vi "Actor Core.vi"(8 "error in":errorcluster, 11 "LF2R IDE in":refnum<class "Main Panel.lvclass">) -> (0 "error out":errorcluster, 3 "Actor out":refnum<class "Actor.lvclass">)   [LabVIEW 2018, in "Main Panel.lvlib" / "Main Panel.lvclass"]
doc: "The user interface for this panel.\n\n----\nPlease see the following web address for additional documentation and tutorial information:\nhttp://www.mooregoodideas.com/mgi-panel-manager/\n\nAuthor: Derek Trepanier\n\nCopyright (c) 2018, Moore Good Ideas, Inc.\n\nAll rights reserved.\n\nRedistribution and use in source and binary forms, with or without modification, are permitted provided that the following conditions are met:\n\n * Redistributions of source code must retain the above copyright notice, this list of conditions and the following disclaimer.\n * Redistributions in binary form must reproduce the above copyright notice, this list of conditions and the following disclaimer in the documentation and/or other materials provided with the distribution.\n * Neither the name of Moore Good Ideas, Inc. nor the names of its contributors may be used to endorse or promote products derived from this software without specific prior written permission.\n\nTHIS SOFTWARE IS PROVIDED BY THE COPYRIGHT HOLDERS AND CONTRIBUTORS \"AS IS\" AND ANY EXPRESS OR IMPLIED WARRANTIES, INCLUDING, BUT NOT LIMITED TO, THE IMPLIED WARRANTIES OF MERCHANTABILITY AND FITNESS FOR A PARTICULAR PURPOSE ARE DISCLAIMED. IN NO EVENT SHALL THE COPYRIGHT OWNER OR CONTRIBUTORS BE LIABLE FOR ANY DIRECT, INDIRECT, INCIDENTAL, SPECIAL, EXEMPLARY, OR CONSEQUENTIAL DAMAGES (INCLUDING, BUT NOT LIMITED TO, PROCUREMENT OF SUBSTITUTE GOODS OR SERVICES; LOSS OF USE, DATA, OR PROFITS; OR BUSINESS INTERRUPTION) HOWEVER CAUSED AND ON ANY THEORY OF LIABILITY, WHETHER IN CONTRACT, STRICT LIABILITY, OR TORT (INCLUDING NEGLIGENCE OR OTHERWISE) ARISING IN ANY WAY OUT OF THE USE OF THIS SOFTWARE, EVEN IF ADVISED OF THE POSSIBILITY OF SUCH DAMAGE."
uses:
  Main Panel.lvclass
  C:/Program Files (x86)/National Instruments/LabVIEW 2018/vi.lib/MGI/Panel Manager/Panel Actor/Panel Actor/Panel Actor.lvclass
  <vilib>/ActorFramework/Actor/Actor.lvclass
  Main Panel.lvclass/Main Panel.ctl
  Const Configuration.ctl
  Const Path Setting.ctl
  Const Image Viewer Setting.ctl
  Framework/Framework/Framework.lvclass
  <vilib>/MGI/Panel Manager/Panel Actor/Panel Actor/Panel Actor.lvclass
  D:/project/hobby/LabVIEW/LF2R/LabVIEW/Source/ScintillaNET/dll/ScintillaNET.dll
  ScintillaNET/dll/ScintillaNET.dll
panel:
  in  "File Path":path
  in  "Script":refnum<k24>(container)
  in  "To Next Frame":bool
  in  "Go to Frame":u16(ring)
  in  "Tab Control":T1(tab)
  in  "WindowsMediaPlayer":refnum<k7>(container)
  in  "basic_state":u16(ring) caption="state" items=["Stand"=0, "Walk"=1, "Run"=2, "Attacking"=3, "Jumping"=4, "Dashing"=5, "Rowing"=6, "Defending"=7, "Defend Broken"=8, "Catching"=9, "Caught"=10, "Injured"=11, "Falling"=12, "Ice"=13, "Lying"=14, "Normal"=15, "Faint"=16, "Drinking"=17, "Burning (Can Attack Teammate)"=18, "Burning Run"=19, "Louis's Special Landing (to frame 94)"=100, "Deep's Special Move (Can Control Up and Down)"=301, "Teleport to the Nearest Teammate"=400, "Teleport to the Nearest Enemy"=401, "Rudolf's Transform"=500, "Rudolf's Transform Back"=501, "Healing"=1700, "Transform to ID (80XX, ID: XX)"=8000, "Transform to LouisEx"=9995, "Message"=9997, "Message Delete"=9998, "Broken Weapon"=9999]
  in  "sound":string
  in  "basic_dvz":i32 caption="dvz"
  in  "basic_dvy":i32 caption="dvy"
  in  "basic_dvx":i32 caption="dvx"
  in  "basic_centery":i32 caption="centery"
  in  "basic_centerx":i32 caption="centerx"
  in  "basic_next":u32 caption="next"
  in  "basic_wait":u32 caption="wait"
  in  "basic_pic":u32 caption="pic"
  in  "basic_mp":i32 caption="mp"
  in  "basic_hit_j":u32 caption="hit_j"
  in  "basic_hit_a":u32 caption="hit_a"
  in  "basic_hit_d":u32 caption="hit_d"
  in  "basic_hit_ja":u32 caption="hit_ja"
  in  "basic_hit_Ua":u32 caption="hit_Ua"
  in  "basic_hit_Fa":u32 caption="hit_Fa"
  in  "basic_hit_Da":u32 caption="hit_Da"
  in  "basic_hit_Dj":u32 caption="hit_Dj"
  in  "basic_hit_Uj":u32 caption="hit_Uj"
  in  "basic_hit_Fj":u32 caption="hit_Fj"
  in  "Sound Play":bool caption="Play"
  in  "bp_y":dbl caption="y"
  in  "bp_x":dbl caption="x"
  in  "w_attacking":u32 caption="attacking"
  in  "w_dvz":i32 caption="dvz"
  in  "w_dvy":i32 caption="dvy"
  in  "w_dvx":i32 caption="dvx"
  in  "w_cover":u32 caption="cover"
  in  "w_weaponact":u32 caption="weaponact"
  in  "w_y":dbl caption="y"
  in  "w_x":dbl caption="x"
  in  "w_kind":u32 caption="kind"
  in  "b_h":u32 caption="h"
  in  "b_w":u32 caption="w"
  in  "b_y":i32 caption="y"
  in  "b_x":i32 caption="x"
  in  "b_kind":u32 caption="kind"
  in  "<b> index":u32(slide) scale=0.0..10.0
  in  "i_zwidth":u32 caption="zwidth"
  in  "i_caughtact 2":u32 caption="caughtact 2"
  in  "i_catchingact 2":u32 caption="catchingact 2"
  in  "i_caughtact 1":u32 caption="caughtact 1"
  in  "i_catchingact 1":u32 caption="catchingact 1"
  in  "i_effect":u32 caption="effect"
  in  "i_injury":i32 caption="injury"
  in  "i_bdefend":i32 caption="bdefend"
  in  "i_vrest":u32 caption="vrest"
  in  "i_arest":u32 caption="arest"
  in  "i_fall":u32 caption="fall"
  in  "i_dvz":i32 caption="dvz"
  in  "i_dvy":i32 caption="dvy"
  in  "i_dvx":i32 caption="dvx"
  in  "i_h":u32 caption="h"
  in  "i_w":u32 caption="w"
  in  "i_y":i32 caption="y"
  in  "i_x":i32 caption="x"
  in  "i_kind":u32 caption="kind"
  in  "<i> index":u32(slide) scale=0.0..10.0
  in  "o_facing":i32 caption="facing"
  in  "o_oid":u32 caption="oid"
  in  "o_action":u32 caption="action"
  in  "o_kind":u32 caption="kind"
  in  "o_x":i32 caption="x"
  in  "o_y":i32 caption="y"
  in  "o_dvx":i32 caption="dvx"
  in  "o_dvy":i32 caption="dvy"
  in  "o_dvz":i32 caption="dvz"
  in  "c_cover":i32 caption="cover"
  in  "c_injury":i32 caption="injury"
  in  "c_dircontrol":i32 caption="dircontrol"
  in  "c_backhurtact":i32 caption="backhurtact"
  in  "c_fronthurtact":i32 caption="fronthurtact"
  in  "c_decrease":i32 caption="decrease"
  in  "c_hurtable":i32 caption="hurtable"
  in  "c_taction":i32 caption="taction"
  in  "c_aaction":i32 caption="aaction"
  in  "c_vaction":i32 caption="vaction"
  in  "c_y":i32 caption="y"
  in  "c_x":i32 caption="x"
  in  "c_kind":u32 caption="kind"
  in  "c_throwvx":i32 caption="throwvx"
  in  "c_throwvy":i32 caption="throwvy"
  in  "c_throwvz":i32 caption="throwvz"
  in  "c_throwinjury":i32 caption="throwinjury"
  in  "title_name":string caption="Name"
  in  "Apply Change":bool
  in  "title_num":u32 caption="Frame Num" format="%03d"
  out "Picture":picture
  out "String":string
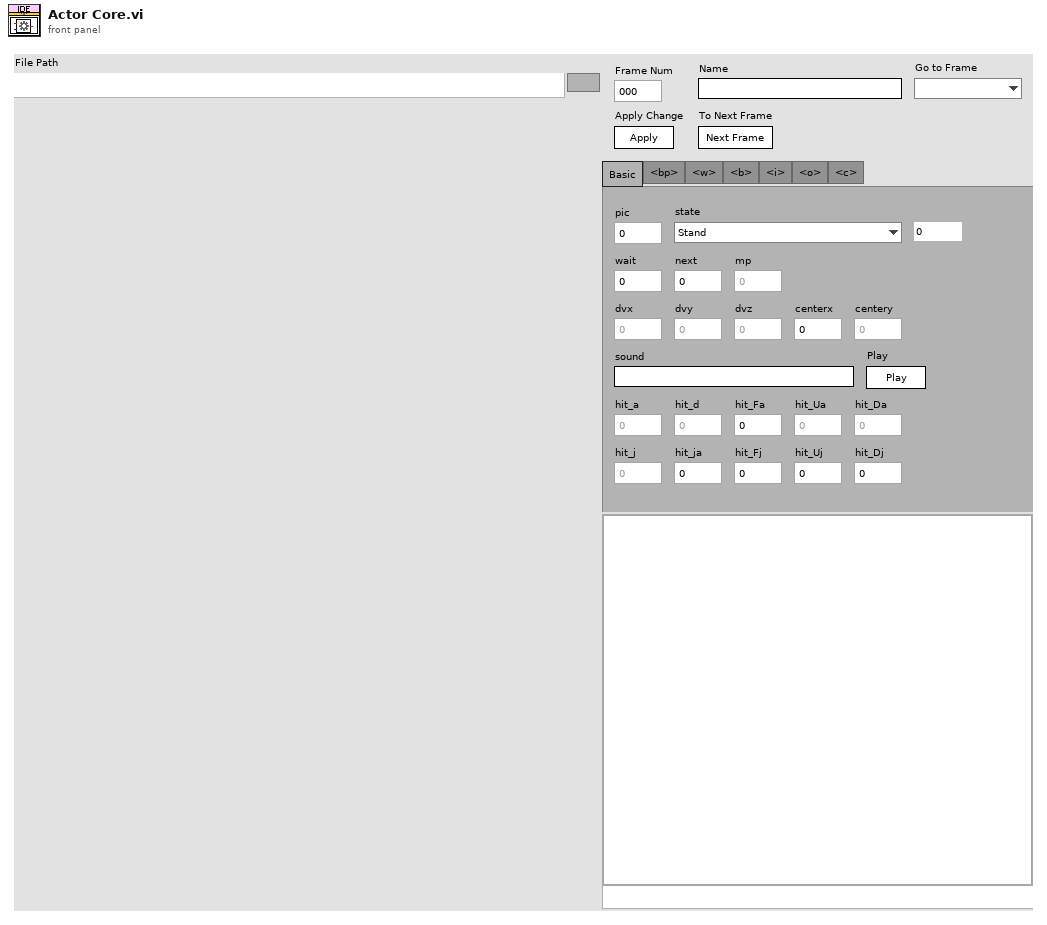
[diagram p1: front panel]
types:
  T1 = enum32{"Basic", "<bp>", "<w>", "<b>", "<i>", "<o>", "<c>"}
  T2 = cluster{"title_num":refnum<vi>, "title_name":refnum<vi>}
  T3 = cluster{"basic_pic":refnum<vi>, "basic_state":refnum<vi>, "basic_wait":refnum<vi>, "basic_next":refnum<vi>}
  T4 = cluster{"basic_centerx":refnum<vi>, "basic_centery":refnum<vi>}
  T5 = cluster{"basic_dvx":refnum<vi>, "basic_dvy":refnum<vi>, "basic_dvz":refnum<vi>}
  T6 = cluster{"b_kind":refnum<vi>, "b_x":refnum<vi>, "b_y":refnum<vi>, "b_w":refnum<vi>, "b_h":refnum<vi>, "<b> index":refnum<vi>}
  T7 = cluster{"w_kind":refnum<vi>, "w_x":refnum<vi>, "w_y":refnum<vi>, "w_weaponact":refnum<vi>, "w_dvx":refnum<vi>, "w_dvy":refnum<vi>, "w_dvz":refnum<vi>, "w_attacking":refnum<vi>, "w_cover":refnum<vi>}
  T8 = cluster{"basic_hit_a":refnum<vi>, "basic_hit_d":refnum<vi>, "basic_hit_j":refnum<vi>, "basic_hit_Fa":refnum<vi>, "basic_hit_Ua":refnum<vi>, "basic_hit_Da":refnum<vi>, "basic_hit_Fj":refnum<vi>, "basic_hit_Uj":refnum<vi>, "basic_hit_Dj":refnum<vi>, "basic_hit_ja":refnum<vi>}
  T9 = cluster{"o_kind":refnum<vi>, "o_x":refnum<vi>, "o_y":refnum<vi>, "o_action":refnum<vi>, "o_dvx":refnum<vi>, "o_dvy":refnum<vi>, "o_dvz":refnum<vi>, "o_oid":refnum<vi>, "o_facing":refnum<vi>}
  T10 = cluster{"i_kind":refnum<vi>, "i_x":refnum<vi>, "i_y":refnum<vi>, "i_w":refnum<vi>, "i_h":refnum<vi>, "i_dvx":refnum<vi>, "i_dvy":refnum<vi>, "i_dvz":refnum<vi>, "i_fall":refnum<vi>, "i_arest":refnum<vi>, "i_vrest":refnum<vi>, "i_bdefend":refnum<vi>, "i_injury":refnum<vi>, "i_zwidth":refnum<vi>, "i_effect":refnum<vi>, "i_catchingact 1":refnum<vi>, "i_catchingact 2":refnum<vi>, "i_caughtact 1":refnum<vi>, "i_caughtact 2":refnum<vi>, "<i> index":refnum<vi>}
  T11 = cluster{"c_kind":refnum<vi>, "c_x":refnum<vi>, "c_y":refnum<vi>, "c_injury":refnum<vi>, "c_cover":refnum<vi>, "c_vaction":refnum<vi>, "c_aaction":refnum<vi>, "c_taction":refnum<vi>, "c_hurtable":refnum<vi>, "c_decrease":refnum<vi>, "c_fronthurtact":refnum<vi>, "c_backhurtact":refnum<vi>, "c_dircontrol":refnum<vi>, "c_throwvx":refnum<vi>, "c_throwvy":refnum<vi>, "c_throwvz":refnum<vi>, "c_throwinjury":refnum<vi>}
  T12 = cluster{"Event Registration Refnum":refnum<event-registration>, "Pnl Actor":refnum<event-registration>}
  T13 = typedef "Main Panel.lvlib/Main Panel.lvclass/Const Configuration.ctl" = cluster{"Language":cluster{"Name":string}, "Path Config":T14, "Image Viewer Config":T15}
  T14 = typedef "Main Panel.lvlib/Main Panel.lvclass/Const Path Setting.ctl" = cluster{"Data Folder Path":path, "PNG Folder Path":path, "mp3 Folder Path":path}
  T15 = typedef "Main Panel.lvlib/Main Panel.lvclass/Const Image Viewer Setting.ctl" = cluster{"Center Point":cluster{"Size":i32, "Color":u32, "Show?":bool}, "bp Point":cluster{"Size":i32, "Color":u32, "Show?":bool}, "w Point":cluster{"Size":i32, "Color":u32, "Show?":bool}, "b Box":cluster{"Fill Color":u32, "Border Color":u32, "Show?":bool}, "i Box":cluster{"Fill Color":u32, "Border Color":u32, "Show?":bool}, "o Point":cluster{"Size":i32, "Color":u32, "Show?":bool}, "c Point":cluster{"Size":i32, "Color":u32, "Show?":bool}}
  T16 = typedef "LF2R IDE.lvlib/LF2R IDE.lvclass/LF2R IDE Cmd.ctl" = enum16{"Save Data File", "Write Configuration", "Save Configuration", "Update Frame Image"}
  T17 = cluster{"Shift":bool, "Ctrl":bool, "Alt":bool, "Cmd":bool, "Opt":bool}
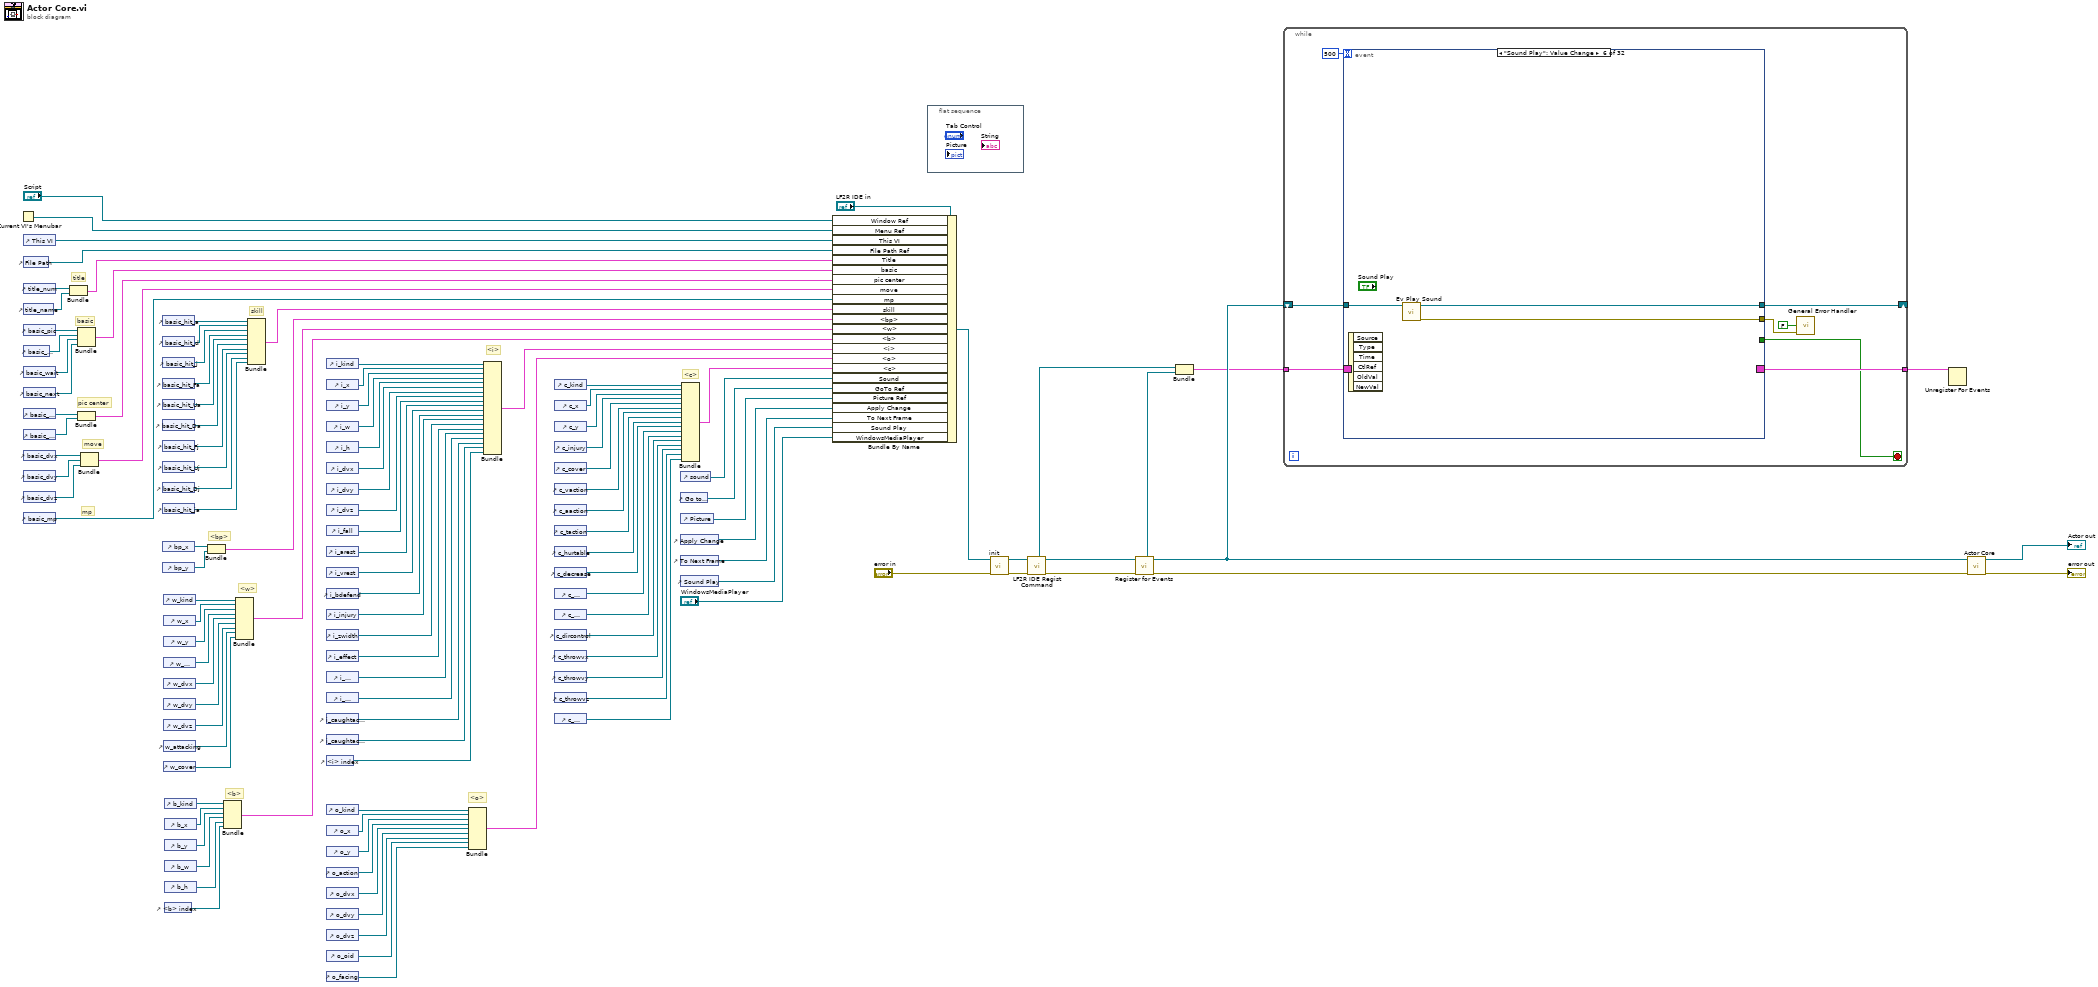
[diagram p0: block diagram]
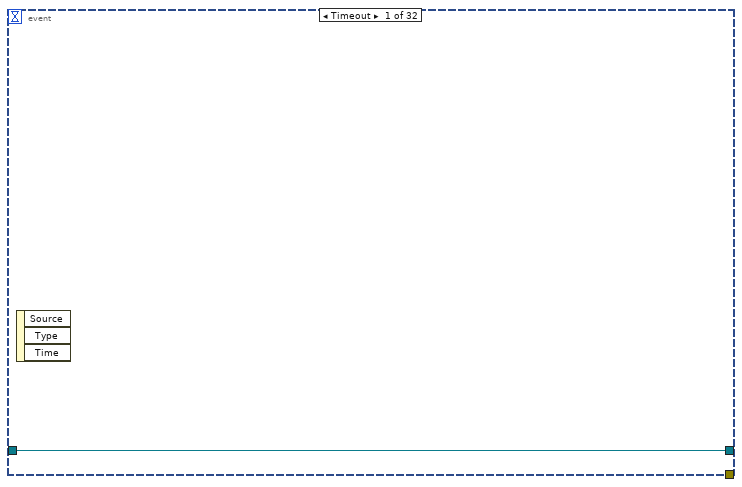
[diagram p2: hidden frame]
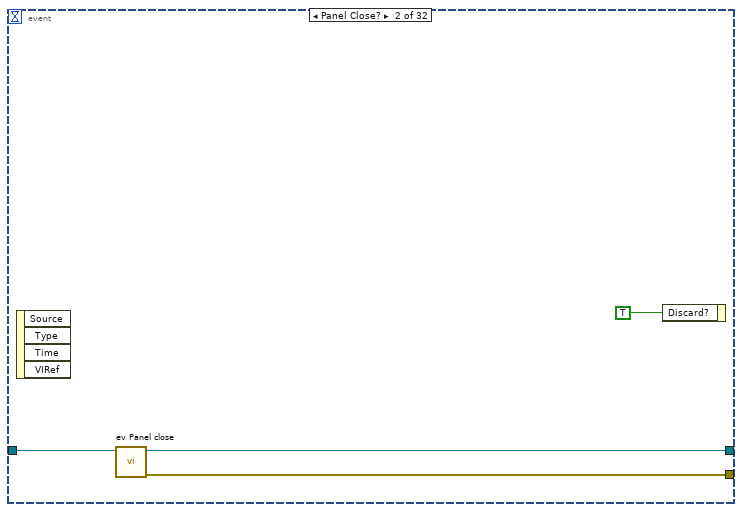
[diagram p3: hidden frame]
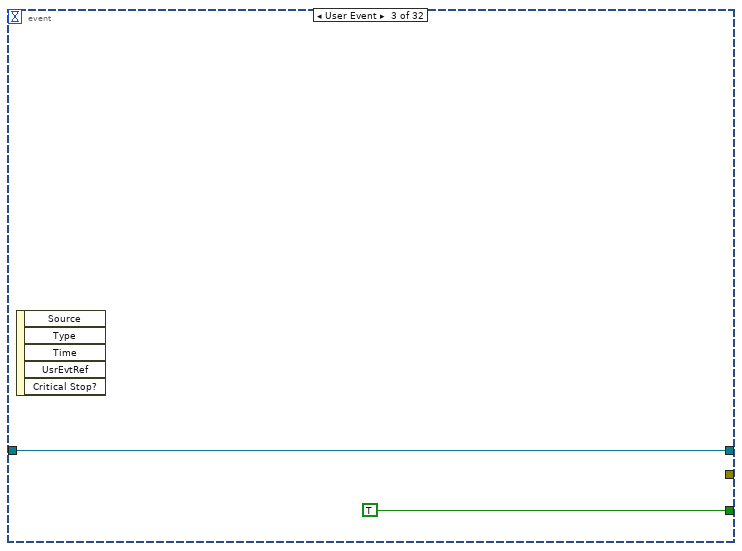
[diagram p4: hidden frame]
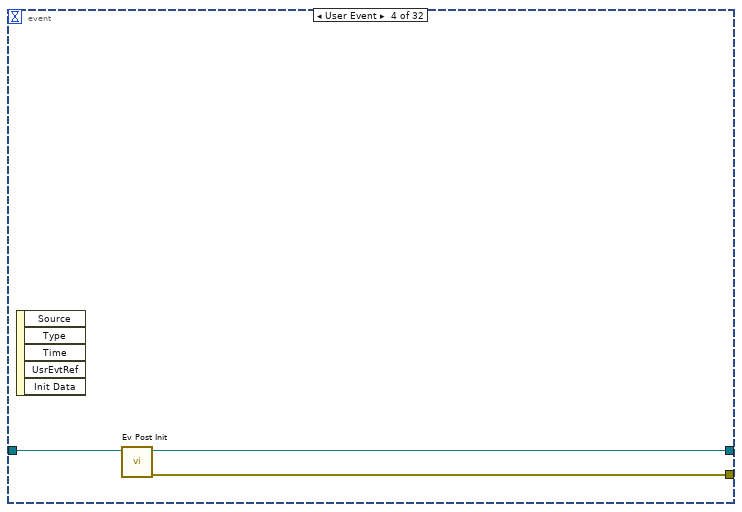
[diagram p5: hidden frame]
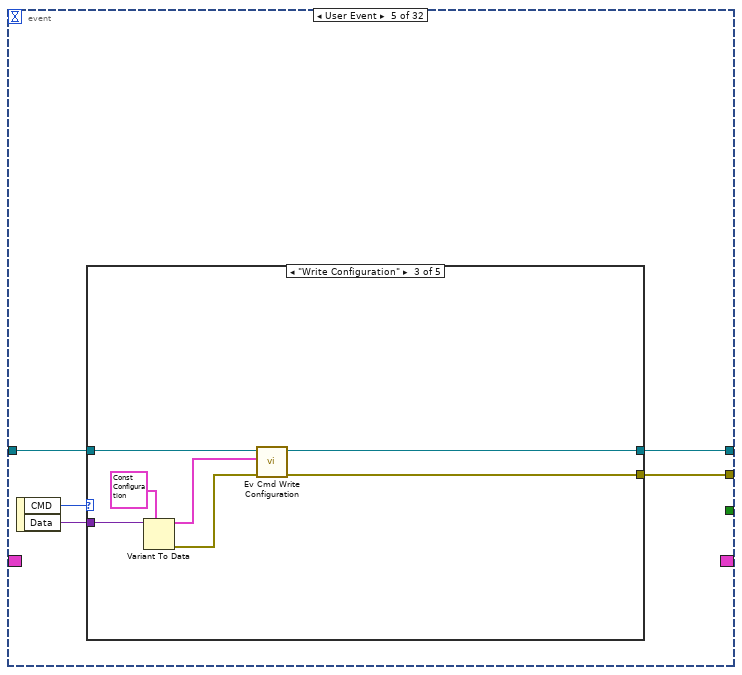
[diagram p6: hidden frame]
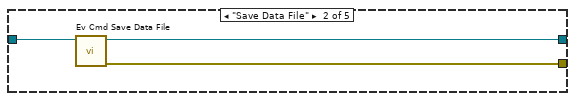
[diagram p8: hidden frame]
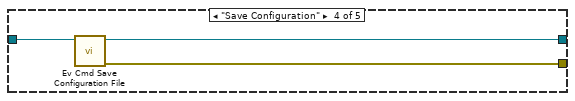
[diagram p9: hidden frame]
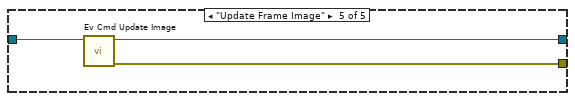
[diagram p10: hidden frame]
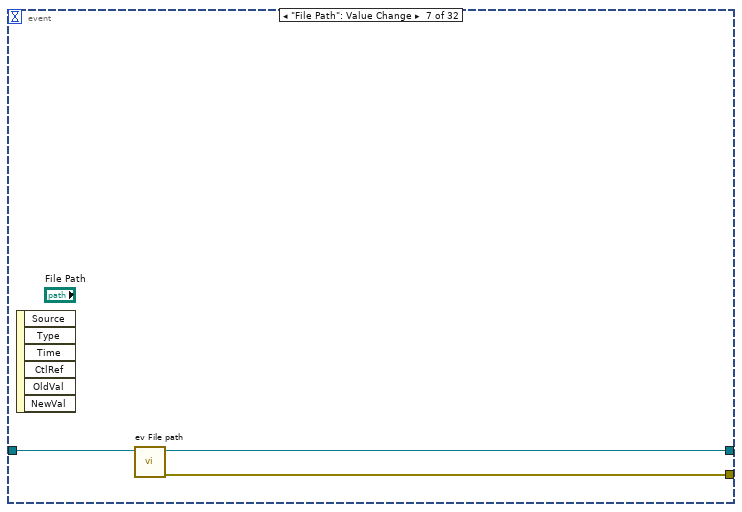
[diagram p11: hidden frame]
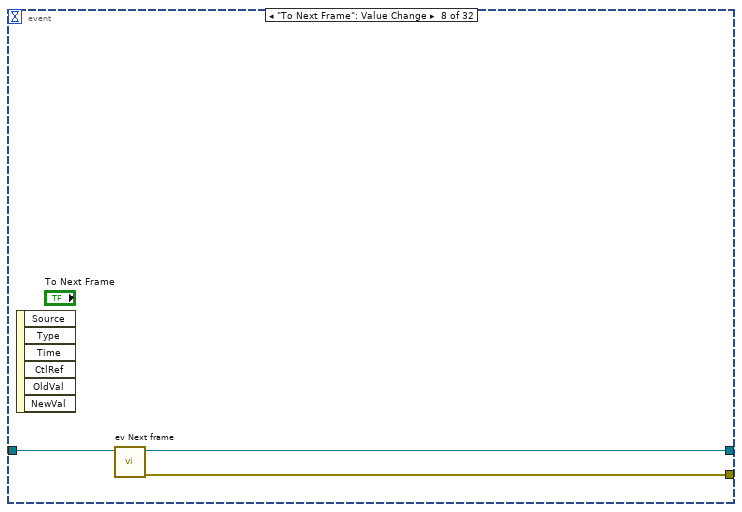
[diagram p12: hidden frame]
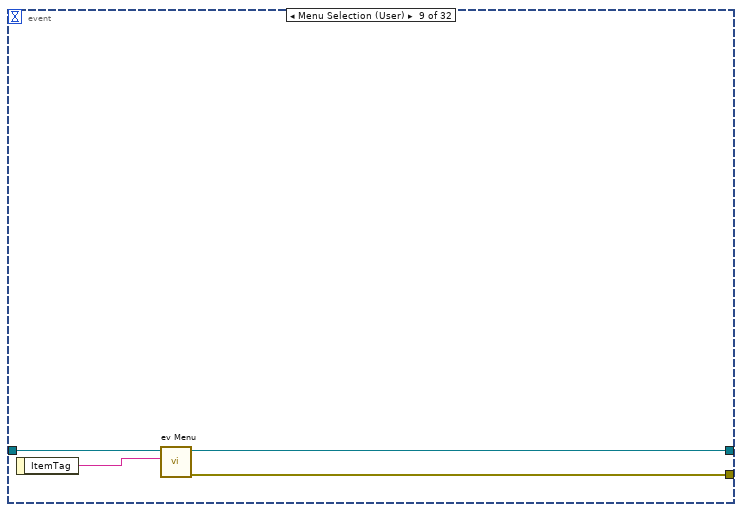
[diagram p13: hidden frame]
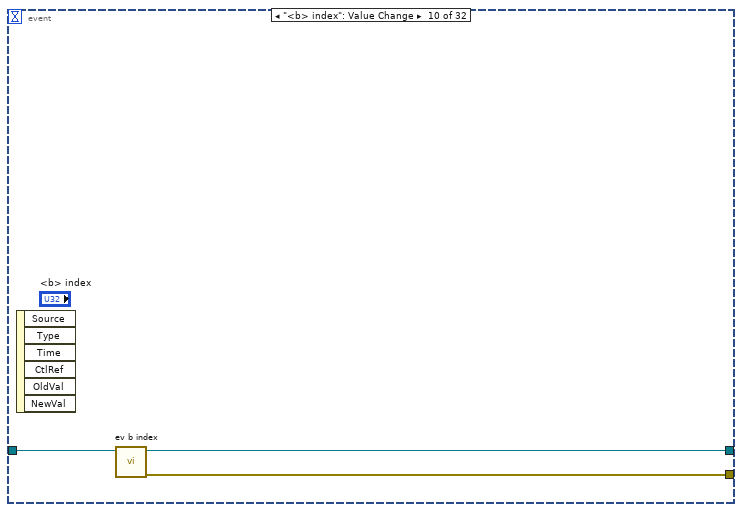
[diagram p14: hidden frame]
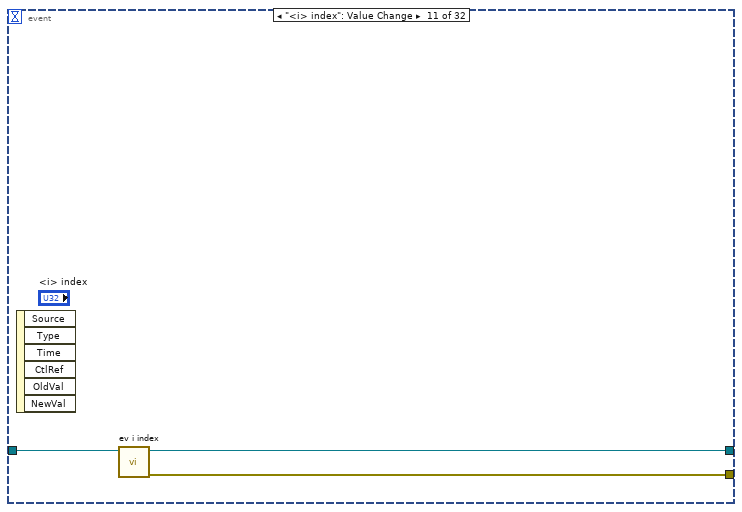
[diagram p15: hidden frame]
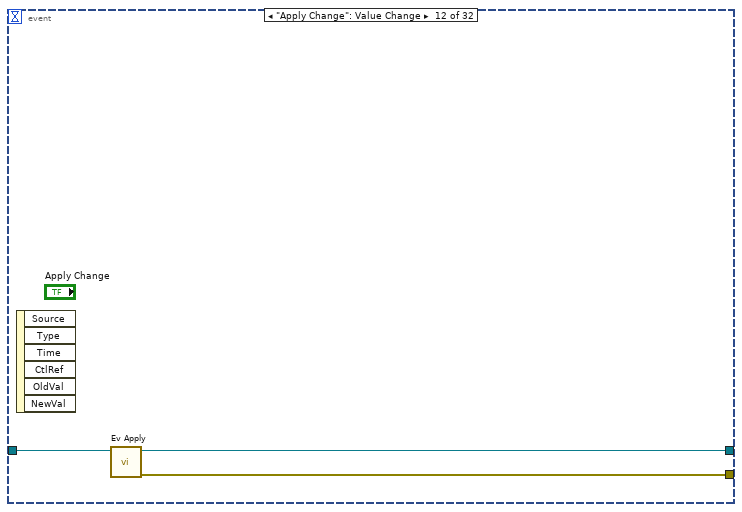
[diagram p16: hidden frame]
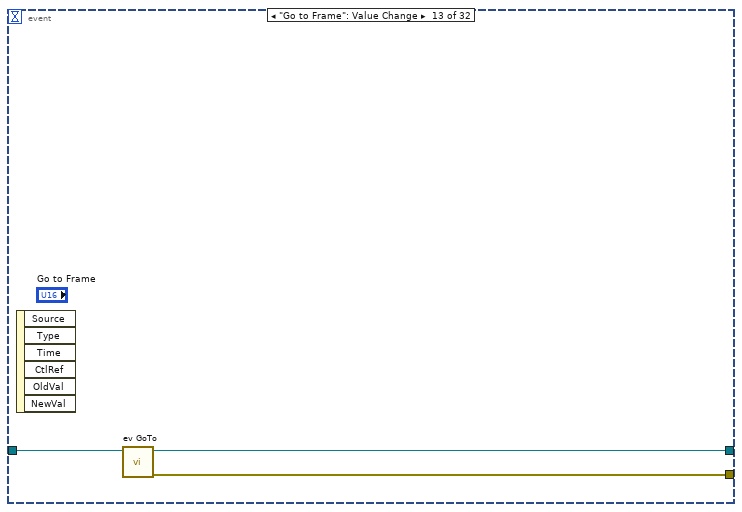
[diagram p17: hidden frame]
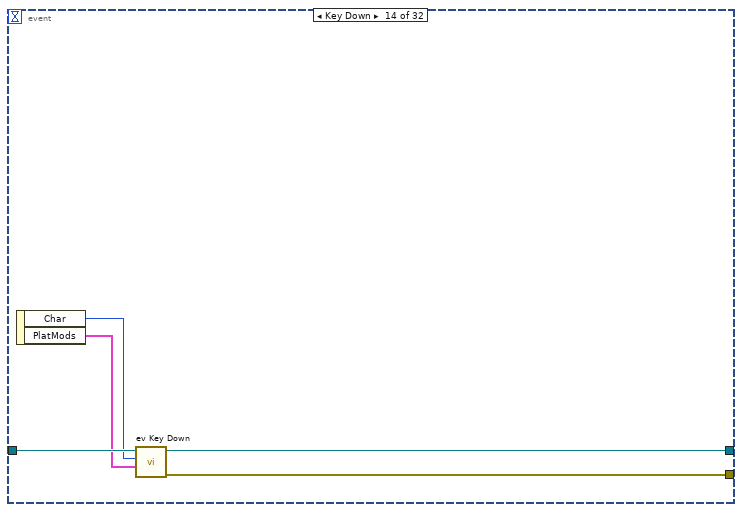
[diagram p18: hidden frame]
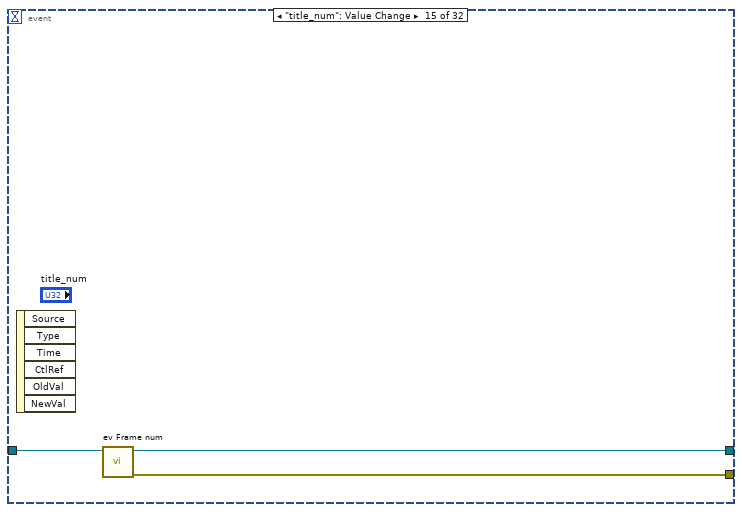
[diagram p19: hidden frame]
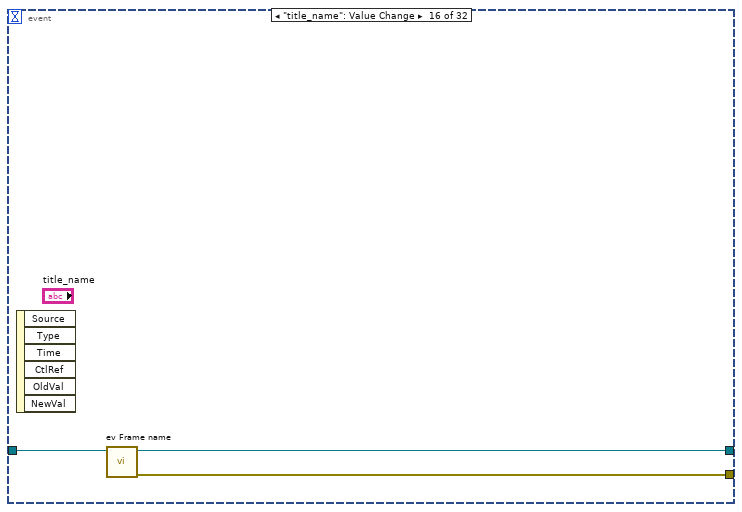
[diagram p20: hidden frame]
diagram:
  # "<c>"
  # "<o>"
  # "<i>"
  # "title"
  # "basic"
  # "pic center"
  # "move"
  # "mp"
  # "skill"
  # "<bp>"
  # "<w>"
  # "<b>"
  n1 = Current VI's Menubar() -> (w22:refnum<k9>)
  n2 = control-ref of="This VI"() -> (w23:refnum<vi>)
  n3 = control-ref of="File Path"() -> (w120:refnum<vi>)
  n4 = control-ref of="title_num"() -> (w111:refnum<vi>)
  n5 = control-ref of="title_name"() -> (w110:refnum<vi>)
  n6 = control-ref of="basic_pic"() -> (w119:refnum<vi>)
  n7 = control-ref of="basic_state"() -> (w4:refnum<vi>)
  n8 = control-ref of="basic_wait"() -> (w118:refnum<vi>)
  n9 = control-ref of="basic_next"() -> (w117:refnum<vi>)
  n10 = control-ref of="basic_centerx"() -> (w116:refnum<vi>)
  n11 = control-ref of="basic_centery"() -> (w115:refnum<vi>)
  n12 = control-ref of="basic_dvx"() -> (w114:refnum<vi>)
  n13 = control-ref of="basic_dvy"() -> (w113:refnum<vi>)
  n14 = control-ref of="basic_dvz"() -> (w112:refnum<vi>)
  n15 = control-ref of="basic_mp"() -> (w105:refnum<vi>)
  n16 = Bundle("title_num"=w111, "title_name"=w110) -> (w109:T2)  [unwired: 1 in]
  n17 = Bundle("basic_pic"=w119, "basic_state"=w4, "basic_wait"=w118, "basic_next"=w117) -> (w108:T3)  [unwired: 1 in]
  n18 = Bundle("basic_centerx"=w116, "basic_centery"=w115) -> (w107:T4)  [unwired: 1 in]
  n19 = Bundle("basic_dvx"=w114, "basic_dvy"=w113, "basic_dvz"=w112) -> (w106:T5)  [unwired: 1 in]
  n20 = control-ref of="basic_hit_a"() -> (w42:refnum<vi>)
  n21 = control-ref of="basic_hit_d"() -> (w41:refnum<vi>)
  n22 = control-ref of="basic_hit_j"() -> (w40:refnum<vi>)
  n23 = control-ref of="basic_hit_Fa"() -> (w39:refnum<vi>)
  n24 = control-ref of="basic_hit_Ua"() -> (w38:refnum<vi>)
  n25 = control-ref of="basic_hit_Da"() -> (w37:refnum<vi>)
  n26 = control-ref of="basic_hit_Fj"() -> (w36:refnum<vi>)
  n27 = control-ref of="basic_hit_Uj"() -> (w35:refnum<vi>)
  n28 = control-ref of="basic_hit_Dj"() -> (w34:refnum<vi>)
  n29 = control-ref of="basic_hit_ja"() -> (w33:refnum<vi>)
  n30 = control-ref of="bp_x"() -> (w31:refnum<vi>)
  n31 = control-ref of="bp_y"() -> (w30:refnum<vi>)
  n32 = control-ref of="w_kind"() -> (w104:refnum<vi>)
  n33 = control-ref of="w_x"() -> (w103:refnum<vi>)
  n34 = control-ref of="w_y"() -> (w102:refnum<vi>)
  n35 = control-ref of="w_weaponact"() -> (w101:refnum<vi>)
  n36 = control-ref of="w_dvx"() -> (w100:refnum<vi>)
  n37 = control-ref of="w_dvy"() -> (w99:refnum<vi>)
  n38 = control-ref of="w_dvz"() -> (w98:refnum<vi>)
  n39 = control-ref of="w_attacking"() -> (w97:refnum<vi>)
  n40 = control-ref of="w_cover"() -> (w29:refnum<vi>)
  n41 = control-ref of="b_kind"() -> (w96:refnum<vi>)
  n42 = control-ref of="b_x"() -> (w95:refnum<vi>)
  n43 = control-ref of="b_y"() -> (w94:refnum<vi>)
  n44 = control-ref of="b_w"() -> (w93:refnum<vi>)
  n45 = control-ref of="b_h"() -> (w92:refnum<vi>)
  n46 = control-ref of="<b> index"() -> (w45:refnum<vi>)
  n47 = Bundle("bp_x"=w31, "bp_y"=w30) -> (w66:cluster{"bp_x":refnum<vi>, "bp_y":refnum<vi>})  [unwired: 1 in]
  n48 = Bundle("b_kind"=w96, "b_x"=w95, "b_y"=w94, "b_w"=w93, "b_h"=w92, "<b> index"=w45) -> (w64:T6)  [unwired: 1 in]
  n49 = Bundle("w_kind"=w104, "w_x"=w103, "w_y"=w102, "w_weaponact"=w101, "w_dvx"=w100, "w_dvy"=w99, "w_dvz"=w98, "w_attacking"=w97, "w_cover"=w29) -> (w65:T7)  [unwired: 1 in]
  n50 = Bundle("basic_hit_a"=w42, "basic_hit_d"=w41, "basic_hit_j"=w40, "basic_hit_Fa"=w39, "basic_hit_Ua"=w38, "basic_hit_Da"=w37, "basic_hit_Fj"=w36, "basic_hit_Uj"=w35, "basic_hit_Dj"=w34, "basic_hit_ja"=w33) -> (w32:T8)  [unwired: 1 in]
  n51 = control-ref of="i_kind"() -> (w91:refnum<vi>)
  n52 = control-ref of="i_x"() -> (w90:refnum<vi>)
  n53 = control-ref of="i_y"() -> (w89:refnum<vi>)
  n54 = control-ref of="i_w"() -> (w88:refnum<vi>)
  n55 = control-ref of="i_h"() -> (w87:refnum<vi>)
  n56 = control-ref of="i_dvx"() -> (w86:refnum<vi>)
  n57 = control-ref of="i_dvy"() -> (w85:refnum<vi>)
  n58 = control-ref of="i_dvz"() -> (w84:refnum<vi>)
  n59 = control-ref of="i_fall"() -> (w83:refnum<vi>)
  n60 = control-ref of="i_arest"() -> (w82:refnum<vi>)
  n61 = control-ref of="i_vrest"() -> (w81:refnum<vi>)
  n62 = control-ref of="i_bdefend"() -> (w80:refnum<vi>)
  n63 = control-ref of="i_injury"() -> (w79:refnum<vi>)
  n64 = control-ref of="i_zwidth"() -> (w28:refnum<vi>)
  n65 = control-ref of="i_effect"() -> (w78:refnum<vi>)
  n66 = control-ref of="i_catchingact 1"() -> (w77:refnum<vi>)
  n67 = control-ref of="i_catchingact 2"() -> (w47:refnum<vi>)
  n68 = control-ref of="i_caughtact 1"() -> (w76:refnum<vi>)
  n69 = control-ref of="i_caughtact 2"() -> (w46:refnum<vi>)
  n70 = control-ref of="<i> index"() -> (w43:refnum<vi>)
  n71 = control-ref of="o_kind"() -> (w75:refnum<vi>)
  n72 = control-ref of="o_x"() -> (w74:refnum<vi>)
  n73 = control-ref of="o_y"() -> (w73:refnum<vi>)
  n74 = control-ref of="o_action"() -> (w72:refnum<vi>)
  n75 = control-ref of="o_dvx"() -> (w71:refnum<vi>)
  n76 = control-ref of="o_dvy"() -> (w70:refnum<vi>)
  n77 = control-ref of="o_dvz"() -> (w69:refnum<vi>)
  n78 = control-ref of="o_oid"() -> (w68:refnum<vi>)
  n79 = control-ref of="o_facing"() -> (w67:refnum<vi>)
  n80 = Bundle("o_kind"=w75, "o_x"=w74, "o_y"=w73, "o_action"=w72, "o_dvx"=w71, "o_dvy"=w70, "o_dvz"=w69, "o_oid"=w68, "o_facing"=w67) -> (w63:T9)  [unwired: 1 in]
  n81 = Bundle("i_kind"=w91, "i_x"=w90, "i_y"=w89, "i_w"=w88, "i_h"=w87, "i_dvx"=w86, "i_dvy"=w85, "i_dvz"=w84, "i_fall"=w83, "i_arest"=w82, "i_vrest"=w81, "i_bdefend"=w80, "i_injury"=w79, "i_zwidth"=w28, "i_effect"=w78, "i_catchingact 1"=w77, "i_catchingact 2"=w47, "i_caughtact 1"=w76, "i_caughtact 2"=w46, "<i> index"=w43) -> (w44:T10)  [unwired: 1 in]
  n82 = control-ref of="c_kind"() -> (w62:refnum<vi>)
  n83 = control-ref of="c_x"() -> (w61:refnum<vi>)
  n84 = control-ref of="c_y"() -> (w60:refnum<vi>)
  n85 = control-ref of="c_injury"() -> (w27:refnum<vi>)
  n86 = control-ref of="c_cover"() -> (w26:refnum<vi>)
  n87 = control-ref of="c_vaction"() -> (w59:refnum<vi>)
  n88 = control-ref of="c_aaction"() -> (w58:refnum<vi>)
  n89 = control-ref of="c_taction"() -> (w57:refnum<vi>)
  n90 = control-ref of="c_hurtable"() -> (w56:refnum<vi>)
  n91 = control-ref of="c_decrease"() -> (w55:refnum<vi>)
  n92 = control-ref of="c_fronthurtact"() -> (w54:refnum<vi>)
  n93 = control-ref of="c_backhurtact"() -> (w53:refnum<vi>)
  n94 = control-ref of="c_dircontrol"() -> (w52:refnum<vi>)
  n95 = control-ref of="c_throwvx"() -> (w51:refnum<vi>)
  n96 = control-ref of="c_throwvy"() -> (w50:refnum<vi>)
  n97 = control-ref of="c_throwvz"() -> (w49:refnum<vi>)
  n98 = control-ref of="c_throwinjury"() -> (w48:refnum<vi>)
  n99 = control-ref of="sound"() -> (w24:refnum<vi>)
  n100 = control-ref of="Go to Frame"() -> (w7:refnum<vi>)
  n101 = control-ref of="Picture"() -> (w1:refnum<vi>)
  n102 = control-ref of="Apply Change"() -> (w6:refnum<vi>)
  n103 = control-ref of="To Next Frame"() -> (w5:refnum<vi>)
  n104 = control-ref of="Sound Play"() -> (w2:refnum<vi>)
  n105 = Bundle("c_kind"=w62, "c_x"=w61, "c_y"=w60, "c_injury"=w27, "c_cover"=w26, "c_vaction"=w59, "c_aaction"=w58, "c_taction"=w57, "c_hurtable"=w56, "c_decrease"=w55, "c_fronthurtact"=w54, "c_backhurtact"=w53, "c_dircontrol"=w52, "c_throwvx"=w51, "c_throwvy"=w50, "c_throwvz"=w49, "c_throwinjury"=w48) -> (w25:T11)  [unwired: 1 in]
  n106 = Bundle By Name(cluster="LF2R IDE in", "Window Ref"="Script", "Menu Ref"=w22, "This VI"=w23, "File Path Ref"=w120, "Title"=w109, "basic"=w108, "pic center"=w107, "move"=w106, "mp"=w105, "skill"=w32, "<bp>"=w66, "<w>"=w65, "<b>"=w64, "<i>"=w44, "<o>"=w63, "<c>"=w25, "Sound"=w24, "GoTo Ref"=w7, "Picture Ref"=w1, "Apply Change"=w6, "To Next Frame"=w5, "Sound Play"=w2, "WindowsMediaPlayer"="WindowsMediaPlayer") -> (w17:refnum<class "Main Panel.lvclass">)
  n107 = flat-sequence {
    frame #0 {
    }
  }
  n108 = call "init.vi"("error in (no error)"="error in", "IDE simple in"=w17) -> ("error out"=w13:errorcluster, "IDE simple out"=w14:refnum<class "Main Panel.lvclass">)  [unwired: 8 in]
  n109 = call "LF2R IDE Regist Command.vi"("error in (no error)"=w13, "LF2R IDE in"=w14) -> ("error out"=w11:errorcluster, "LF2R IDE out"=w12:refnum<class "Main Panel.lvclass">, "Event Registration Refnum"=w10:refnum<event-registration>)  [unwired: 7 in]
  n110 = call <vilib>:"Register for Events.vi"("Error In"=w11, "Panel Actor in"=w12) -> ("Error Out"=w20:errorcluster, "Panel Actor out"=w19:refnum<class "Main Panel.lvclass">, "Pnl Actor"=w9:refnum<event-registration>)  [unwired: 6 in, 1 out]
  n111 = Bundle("Event Registration Refnum"=w10, "Pnl Actor"=w9) -> (w8:T12)  [unwired: 1 in]
  n112 = while {
    shift-right: [w129] -> _
    shift-left: w19 -> [w130]
    tunnel: [w128] -> w18
    tunnel: w8 -> [w126]
    stop <- w125 stop-if-true
    n113 = event shown="[5] \"Sound Play\": Value Change" {
      selector: w126 -> [_ _ _ _ _ _ _ _ _ _ _ _ _ _ _ _ _ _ _ _ _ _ _ _ _ _ _ _ _ _ _ _]
      dyn-events: [_ _ _ _ _ _ _ _ _ _ _ _ _ _ _ _ _ _ _ _ _ _ _ _ _ _ _ _ _ _ _ _] -> w128
      timeout: 500 -> [_ _ _ _ _ _ _ _ _ _ _ _ _ _ _ _ _ _ _ _ _ _ _ _ _ _ _ _ _ _ _ _]
      tunnel: w130 -> [w131 w134 w137 w140 w144 w165 w168 w171 w175 w178 w181 w184 w187 w192 w195 w198 w201 w203 w207 w210 w213 w214 w219 w221 w225 w226 w231 w233 w237 w238 w243 w245]
      tunnel: [w131 w132 w137 w139 w143 w163 w166 w170 w174 w177 w180 w183 w185 w190 w193 w197 w200 w203 w207 w208 w212 w214 w218 w221 w223 w226 w229 w233 w236 w238 w241 w245] -> w129
      tunnel: [_ _ TRUE ("Stop") _ _ _ _ _ _ _ _ _ _ _ _ _ _ _ _ _ _ _ _ _ _ _ _ _ _ _ _ _] -> w125
      tunnel: [_ w133 _ w138 w141 w164 w167 w169 w173 w176 w179 w182 w186 w191 w194 w196 w199 w204 w205 w209 w211 w215 w217 w220 w224 w227 w230 w232 w235 w239 w242 w244] -> w124
      event Timeout {
        n114 = event-data() -> ()  [unwired: 1 in, 3 out]
      }
      event Panel Close? {
        n115 = event-data() -> ()  [unwired: 1 in, 4 out]
        n116 = call "ev Panel close.vi"("LF2R IDE in"=w134) -> ("error out"=w133:errorcluster, "LF2R IDE out"=w132:refnum<class "Main Panel.lvclass">)  [unwired: 9 in]
        n117 = event-data("Discard?"=TRUE) -> ()  [unwired: 1 in, 1 out]
      }
      event User Event {
        n118 = event-data() -> ()  [unwired: 1 in, 5 out]
      }
      event User Event {
        n119 = event-data() -> ()  [unwired: 1 in, 5 out]
        n120 = call "Ev Post Init.vi"("LF2R IDE in"=w140) -> ("error out"=w138:errorcluster, "LF2R IDE out"=w139:refnum<class "Main Panel.lvclass">)  [unwired: 9 in]
      }
      event User Event {
        n121 = event-data() -> ("CMD"=w145:T16, "Data"=w142:variant)  [unwired: 1 in]
        n122 = case shown="\"Write Configuration\"" w145 {
          tunnel: w144 -> [w146 w149 w156 w159 w162]
          tunnel: [w146 w148 w154 w157 w161] -> w143
          tunnel: w142 -> [_ _ w153 _ _]
          tunnel: [_ w147 w155 w158 w160] -> w141
          frame Default {
          }
          frame "Save Data File" {
            n123 = call "Ev Cmd Save Data File.vi"("LF2R IDE in"=w149) -> ("error out"=w147:errorcluster, "LF2R IDE out"=w148:refnum<class "Main Panel.lvclass">)  [unwired: 9 in]
          }
          frame "Write Configuration" {
            n124 = Variant To Data(type=T13 {"Language"={"Name"=""}, "Path Config"={"Data Folder Path"=path "", "PNG Folder Path"=path "", "mp3 Folder Path"=path ""}, "Image Viewer Config"={"Center Point"={"Size"=3, "Color"=0, "Show?"=FALSE}, "bp Point"={"Size"=3, "Color"=0, "Show?"=FALSE}, "w Point"={"Size"=3, "Color"=0, "Show?"=FALSE}, "b Box"={"Fill Color"=0, "Border Color"=0, "Show?"=FALSE}, "i Box"={"Fill Color"=0, "Border Color"=0, "Show?"=FALSE}, "o Point"={"Size"=3, "Color"=0, "Show?"=FALSE}, "c Point"={"Size"=3, "Color"=0, "Show?"=FALSE}}} ("Configuration"), Variant=w153) -> (data=w151:T13, error out=w150:errorcluster)  [unwired: 1 in]
            n125 = call "Ev Cmd Write Configuration.vi"("error in (no error)"=w150, "Configuration"=w151, "LF2R IDE in"=w156) -> ("error out"=w155:errorcluster, "LF2R IDE out"=w154:refnum<class "Main Panel.lvclass">)  [unwired: 7 in]
          }
          frame "Save Configuration" {
            n126 = call "Ev Cmd Save Configuration File.vi"("LF2R IDE in"=w159) -> ("error out"=w158:errorcluster, "LF2R IDE out"=w157:refnum<class "Main Panel.lvclass">)  [unwired: 9 in]
          }
          frame "Update Frame Image" {
            n127 = call "Ev Cmd Update Image.vi"("LF2R IDE in"=w162) -> ("error out"=w160:errorcluster, "LF2R IDE out"=w161:refnum<class "Main Panel.lvclass">)  [unwired: 9 in]
          }
        }
      }
      event "Sound Play": Value Change {
        n128 = event-data() -> ()  [unwired: 1 in, 6 out]
        n129 = call "Ev Play Sound.vi"("Main Panel in"=w165) -> ("error out"=w164:errorcluster, "Main Panel out"=w163:refnum<class "Main Panel.lvclass">)  [unwired: 9 in]
      }
      event "File Path": Value Change {
        n130 = event-data() -> ()  [unwired: 1 in, 6 out]
        n131 = call "ev File path.vi"("LF2R IDE in"=w168) -> ("error out"=w167:errorcluster, "LF2R IDE out"=w166:refnum<class "Main Panel.lvclass">)  [unwired: 9 in]
      }
      event "To Next Frame": Value Change {
        n132 = event-data() -> ()  [unwired: 1 in, 6 out]
        n133 = call "ev Next frame.vi"("IDE simple in"=w171) -> ("error out"=w169:errorcluster, "IDE simple out"=w170:refnum<class "Main Panel.lvclass">)  [unwired: 9 in]
      }
      event Menu Selection (User) {
        n134 = event-data() -> ("ItemTag"=w172:string)  [unwired: 1 in]
        n135 = call "ev Menu.vi"("ItemTag"=w172, "LF2R IDE in"=w175) -> ("error out"=w173:errorcluster, "LF2R IDE out"=w174:refnum<class "Main Panel.lvclass">)  [unwired: 8 in]
      }
      event "<b> index": Value Change {
        n136 = event-data() -> ()  [unwired: 1 in, 6 out]
        n137 = call "ev b index.vi"("IDE simple in"=w178) -> ("error out"=w176:errorcluster, "IDE simple out"=w177:refnum<class "Main Panel.lvclass">)  [unwired: 9 in]
      }
      event "<i> index": Value Change {
        n138 = event-data() -> ()  [unwired: 1 in, 6 out]
        n139 = call "ev i index.vi"("IDE simple in"=w181) -> ("error out"=w179:errorcluster, "IDE simple out"=w180:refnum<class "Main Panel.lvclass">)  [unwired: 9 in]
      }
      event "Apply Change": Value Change {
        n140 = event-data() -> ()  [unwired: 1 in, 6 out]
        n141 = call "Ev Apply.vi"("IDE simple in"=w184) -> ("error out"=w182:errorcluster, "IDE simple out"=w183:refnum<class "Main Panel.lvclass">)  [unwired: 9 in]
      }
      event "Go to Frame": Value Change {
        n142 = event-data() -> ()  [unwired: 1 in, 6 out]
        n143 = call "ev GoTo.vi"("LF2R IDE in"=w187) -> ("error out"=w186:errorcluster, "LF2R IDE out"=w185:refnum<class "Main Panel.lvclass">)  [unwired: 9 in]
      }
      event Key Down {
        n144 = event-data() -> ("Char"=w189:i16, "PlatMods"=w188:T17)  [unwired: 1 in]
        n145 = call "ev Key Down.vi"("PlatMods"=w188, "Char"=w189, "LF2R IDE in"=w192) -> ("error out"=w191:errorcluster, "LF2R IDE out"=w190:refnum<class "Main Panel.lvclass">)  [unwired: 7 in]
      }
      event "title_num": Value Change {
        n146 = event-data() -> ()  [unwired: 1 in, 6 out]
        n147 = call "ev Frame num.vi"("IDE simple in"=w195) -> ("error out"=w194:errorcluster, "IDE simple out"=w193:refnum<class "Main Panel.lvclass">)  [unwired: 9 in]
      }
      event "title_name": Value Change {
        n148 = event-data() -> ()  [unwired: 1 in, 6 out]
        n149 = call "ev Frame name.vi"("LF2R IDE in"=w198) -> ("error out"=w196:errorcluster, "LF2R IDE out"=w197:refnum<class "Main Panel.lvclass">)  [unwired: 9 in]
      }
      event "basic_pic", "basic_wait", "basic_next", "basic_dvx", "basic_dvy", "basic_dvz", "basic_centerx", "basic_centery", "basic_hit_Fa", "basic_hit_Fj", "basic_hit_Ua", "basic_hit_Uj", "basic_hit_Dj", "basic_hit_ja", "basic_hit_d", "basic_hit_a", "basic_hit_j", "basic_hit_Da", "basic_mp", "basic_state": Value Change {
        n150 = event-data() -> ()  [unwired: 1 in, 6 out]
        n151 = flat-sequence {
          frame #0 {
            # "basic"
          }
        }
        n152 = call "Ev Basic Data.vi"("IDE simple in"=w201) -> ("error out"=w199:errorcluster, "IDE simple out"=w200:refnum<class "Main Panel.lvclass">)  [unwired: 9 in]
      }
      event "basic_pic", "basic_wait", "basic_next", "basic_centerx", "basic_centery", "basic_dvx", "basic_dvy", "basic_dvz", "basic_mp", "basic_hit_Fa", "basic_hit_Fj", "basic_hit_Ua", "basic_hit_Uj", "basic_hit_Dj", "basic_hit_ja", "basic_hit_d", "basic_hit_a", "basic_hit_j", "basic_hit_Da": Key Down {
        n153 = event-data() -> ("CtlRef"=w202:refnum<vi>)  [unwired: 1 in]
        n154 = call "Num Ref Update Color.vi"("Num ref"=w202) -> ("error out"=w204:errorcluster)  [unwired: 10 in]
      }
      event "basic_state": Key Down {
        n155 = event-data() -> ("CtlRef"=w206:refnum<vi>)  [unwired: 1 in]
        n156 = call "Ring Ref Update Color.vi"("Num ref"=w206) -> ("error out"=w205:errorcluster)  [unwired: 10 in]
      }
      event "sound": Value Change {
        n157 = event-data() -> ()  [unwired: 1 in, 1 out]
        n158 = call "Ev Sound.vi"("IDE simple in"=w210) -> ("error out"=w209:errorcluster, "IDE simple out"=w208:refnum<class "Main Panel.lvclass">)  [unwired: 9 in]
      }
      event "bp_x", "bp_y": Value Change {
        n159 = event-data() -> ()  [unwired: 1 in, 6 out]
        n160 = flat-sequence {
          frame #0 {
            # "<bp>"
          }
        }
        n161 = call "Ev bp.vi"("IDE simple in"=w213) -> ("error out"=w211:errorcluster, "IDE simple out"=w212:refnum<class "Main Panel.lvclass">)  [unwired: 9 in]
      }
      event "bp_x", "bp_y": Key Down {
        n162 = event-data() -> ("CtlRef"=w216:refnum<vi>)  [unwired: 1 in]
        n163 = call "Num Ref Update Color.vi"("Num ref"=w216) -> ("error out"=w215:errorcluster)  [unwired: 10 in]
      }
      event "w_kind", "w_x", "w_y", "w_weaponact", "w_cover", "w_dvx", "w_dvy", "w_dvz", "w_attacking": Value Change {
        n164 = event-data() -> ()  [unwired: 1 in, 6 out]
        n165 = flat-sequence {
          frame #0 {
            # "<w>"
          }
        }
        n166 = call "Ev w.vi"("IDE simple in"=w219) -> ("error out"=w217:errorcluster, "IDE simple out"=w218:refnum<class "Main Panel.lvclass">)  [unwired: 9 in]
      }
      event "w_kind", "w_x", "w_y", "w_weaponact", "w_cover", "w_dvx", "w_dvy", "w_dvz", "w_attacking": Key Down {
        n167 = event-data() -> ("CtlRef"=w222:refnum<vi>)  [unwired: 1 in]
        n168 = call "Num Ref Update Color.vi"("Num ref"=w222) -> ("error out"=w220:errorcluster)  [unwired: 10 in]
      }
      event "b_kind", "b_x", "b_y", "b_w", "b_h": Value Change {
        n169 = event-data() -> ()  [unwired: 1 in, 6 out]
        n170 = flat-sequence {
          frame #0 {
            # "<b>"
          }
        }
        n171 = call "Ev b.vi"("IDE simple in"=w225) -> ("error out"=w224:errorcluster, "IDE simple out"=w223:refnum<class "Main Panel.lvclass">)  [unwired: 9 in]
      }
      event "b_kind", "b_x", "b_y", "b_w", "b_h": Key Down {
        n172 = event-data() -> ("CtlRef"=w228:refnum<vi>)  [unwired: 1 in]
        n173 = call "Num Ref Update Color.vi"("Num ref"=w228) -> ("error out"=w227:errorcluster)  [unwired: 10 in]
      }
      event "i_kind", "i_x", "i_y", "i_w", "i_h", "i_dvx", "i_dvy", "i_dvz", "i_fall", "i_arest", "i_vrest", "i_bdefend", "i_injury", "i_effect", "i_catchingact 1", "i_caughtact 1", "i_catchingact 2", "i_caughtact 2", "i_zwidth": Value Change {
        n174 = event-data() -> ()  [unwired: 1 in, 6 out]
        n175 = flat-sequence {
          frame #0 {
            # "<i>"
          }
        }
        n176 = call "Ev i.vi"("IDE simple in"=w231) -> ("error out"=w230:errorcluster, "IDE simple out"=w229:refnum<class "Main Panel.lvclass">)  [unwired: 9 in]
      }
      event "i_kind", "i_x", "i_y", "i_w", "i_h", "i_dvx", "i_dvy", "i_dvz", "i_fall", "i_arest", "i_vrest", "i_bdefend", "i_injury", "i_effect", "i_catchingact 1", "i_caughtact 1", "i_catchingact 2", "i_caughtact 2", "i_zwidth": Key Down {
        n177 = event-data() -> ("CtlRef"=w234:refnum<vi>)  [unwired: 1 in]
        n178 = call "Num Ref Update Color.vi"("Num ref"=w234) -> ("error out"=w232:errorcluster)  [unwired: 10 in]
      }
      event "o_kind", "o_x", "o_y", "o_dvx", "o_dvy", "o_dvz", "o_action", "o_oid", "o_facing": Value Change {
        n179 = event-data() -> ()  [unwired: 1 in, 1 out]
        n180 = flat-sequence {
          frame #0 {
            # "<o>"
          }
        }
        n181 = call "Ev o.vi"("IDE simple in"=w237) -> ("error out"=w235:errorcluster, "IDE simple out"=w236:refnum<class "Main Panel.lvclass">)  [unwired: 9 in]
      }
      event "o_kind", "o_x", "o_y", "o_dvx", "o_dvy", "o_dvz", "o_action", "o_oid", "o_facing": Key Down {
        n182 = event-data() -> ("CtlRef"=w240:refnum<vi>)  [unwired: 1 in]
        n183 = call "Num Ref Update Color.vi"("Num ref"=w240) -> ("error out"=w239:errorcluster)  [unwired: 10 in]
      }
      event "c_kind", "c_x", "c_y", "c_vaction", "c_aaction", "c_taction", "c_hurtable", "c_decrease", "c_fronthurtact", "c_backhurtact", "c_dircontrol", "c_throwvx", "c_throwvy", "c_throwvz", "c_throwinjury", "c_injury", "c_cover": Value Change {
        n184 = event-data() -> ()  [unwired: 1 in, 1 out]
        n185 = flat-sequence {
          frame #0 {
            # "<c>"
          }
        }
        n186 = call "Ev c.vi"("IDE simple in"=w243) -> ("error out"=w242:errorcluster, "IDE simple out"=w241:refnum<class "Main Panel.lvclass">)  [unwired: 9 in]
      }
      event "c_kind", "c_x", "c_y", "c_vaction", "c_aaction", "c_taction", "c_hurtable", "c_decrease", "c_fronthurtact", "c_backhurtact", "c_dircontrol", "c_throwvx", "c_throwvy", "c_throwvz", "c_throwinjury", "c_injury", "c_cover": Key Down {
        n187 = event-data() -> ("CtlRef"=w246:refnum<vi>)  [unwired: 1 in]
        n188 = call "Num Ref Update Color.vi"("Num ref"=w246) -> ("error out"=w244:errorcluster)  [unwired: 10 in]
      }
    }
    n189 = call <vilib>:"General Error Handler.vi"("search ni.com link visible?(T)"=FALSE, "error in (no error)"=w124) -> ()  [unwired: 9 in, 5 out]
  }
  n190 = Unregister For Events(event registration refnum=w18) -> ()  [unwired: 1 in, 1 out]
  n191 = call-parent "Actor Core.vi"("error in"=w20, "Panel Actor in"=w19) -> ("error out"=→"error out":errorcluster, "Actor out"=→"Actor out":refnum<class "Actor.lvclass">)  [unwired: 8 in]
